vi "PH_IEEE1394Camera.evt call SetTimeout.vi"(0 "i ref in":refnum<vi>, 2 "Instance":string, 3 "TO [ms]":u32, 5 "error in (no error)":errorcluster) -> (14 "i ref out":refnum<vi>, 19 "error out":errorcluster)   [LabVIEW 2014, in "PH_IEEE1394Camera.lvlib"]
doc: "This VI sends a simple call for SetTimeout."
uses:
  PH_IEEE1394Camera.lvlib
  CS_Core/CSSystem/CoreLib/CoreLib.int 2 byte array.vi
  CS_Core/CSSystem/CoreLib/CoreLib.lvlib
  CS_Core/BaseProcess/BaseProcess.lvlib
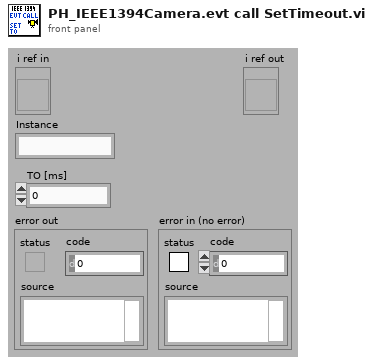
[diagram p1: front panel]
types:
  T1 = typedef "CoreDefs.rawDataType.ctl" = i8[]
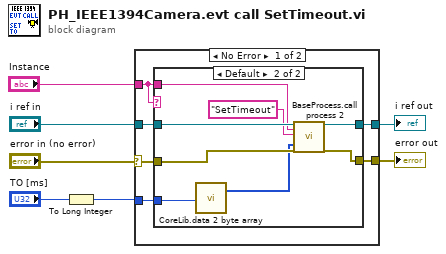
[diagram p0: block diagram]
diagram:
  n1 = To Long Integer(number="TO [ms]") -> (32bit integer=w1:i32)
  n2 = case shown="No Error" "error in (no error)" {
    selector: "error in (no error)" -> [w10 w24]
    tunnel: [w13 w25] -> w5
    tunnel: [w12 w24] -> w4
    tunnel: "i ref in" -> [w11 w25]
    tunnel: "Instance" -> [w9 _]
    tunnel: w1 -> [w8 _]
    frame No Error {
      n3 = case shown="Default" w9 {
        tunnel: [w15 w23] -> w13
        tunnel: [w14 w22] -> w12
        tunnel: w11 -> [w15 w21]
        tunnel: w9 -> [_ w20]
        tunnel: w10 -> [w14 w18]
        tunnel: w8 -> [_ w16]
        frame "N/A" {
        }
        frame Default {
          n4 = call-poly "CoreLib.data 2 byte array.vi"("i32"=w16) -> ("byteArray out"=w17:T1)  [unwired: 18 in]
          n5 = call "BaseProcess.call process 2.vi"("i ref in"=w21, "Object"=w20, "Selector"="SetTimeout", "Data"=w17, "error in (no error)"=w18) -> ("i ref out"=w23:refnum<vi>, "error out"=w22:errorcluster)  [unwired: 13 in]
        }
      }
    }
    frame Error {
    }
  }
  "error out" <- w4
  "i ref out" <- w5
